vi "Stop Point.vi"(5 "Series Enqueuer":refnum<class "Message Enqueuer.lvclass">, 7 "Task-Point Ident":string, 8 "error in":errorcluster, 11 "MSS in":refnum<class "Measure and Stimulus Subsystems.lvclass">) -> (0 "error out":errorcluster, 3 "MSS out":refnum<class "Measure and Stimulus Subsystems.lvclass">)   [LabVIEW 2023, in "HAL GOOP4.lvlib" / "Measure and Stimulus Subsystems.lvclass"]
uses:
  Measure and Stimulus Subsystems.lvclass
  <vilib>/ActorFramework/Message Enqueuer/Message Enqueuer.lvclass
  Measure and Stimulus Subsystems.lvclass/Measure and Stimulus Subsystems.ctl
  Series/ISeries Actor/ISeries Actor Messages/Stop Point on Target Msg/Stop Point on Target Msg.lvclass/Stop Point on Target Msg.ctl
  <vilib>/ActorFramework/Message Enqueuer/Message Enqueuer.lvclass/Message Enqueuer.ctl
  <vilib>/ActorFramework/Message Enqueuer/Enqueue.vi
  Series/ISeries Actor/ISeries Actor Messages/Stop Point on Target Msg/Stop Point on Target Msg.lvclass
  <vilib>/Utility/LVClass/Get LV Class Name.vi
  <resource>/AFDebug/Generate Trace for Message.vi
  <vilib>/ActorFramework/Message Priority Queue/Priority Enqueue.vi
  Virt Instr Host/Virt Instr Local.lvclass
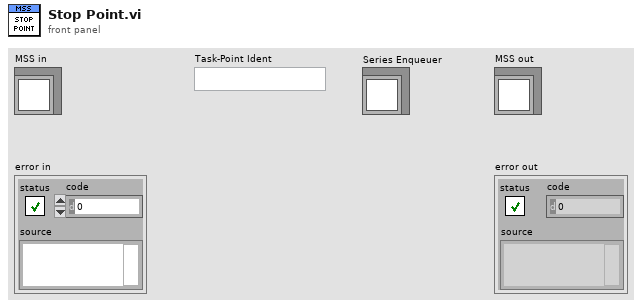
[diagram p1: front panel]
types:
  T1 = map{string, refnum<class "Virt Instr Local.lvclass">}
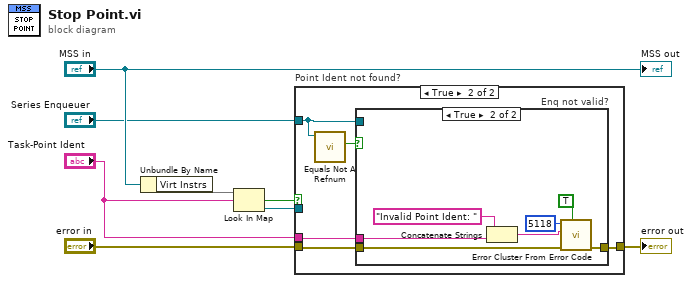
[diagram p0: block diagram]
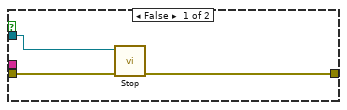
[diagram p2: hidden frame]
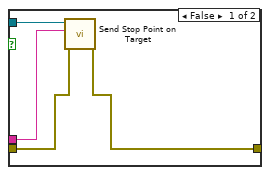
[diagram p3: hidden frame]
diagram:
  n1 = Unbundle By Name("MSS in") -> ("Virt Instrs"=w7:T1)
  n2 = Look In Map(map=w7, key="Task-Point Ident") -> (key not found?=w6:bool, value=w5:refnum<class "Virt Instr Local.lvclass">)  [unwired: 1 in]
  n3 = case "Point Ident not found?" shown="True" w6 {
    tunnel: w5 -> [w10 _]
    tunnel: "error in" -> [w9 w16]
    tunnel: [w11 w15] -> w4
    tunnel: "Series Enqueuer" -> [_ w12]
    tunnel: "Task-Point Ident" -> [_ w14]
    frame False {
      n4 = call-dynamic "Stop.vi"("error in (no error)"=w9, "Virt Instr Base in"=w10) -> ("error out"=w11:errorcluster)  [unwired: 8 in, 1 out]
    }
    frame True {
      n5 = call <vilib>:"Equals Not A Refnum.vi"("Message Enqueuer"=w12) -> ("Not a refnum?"=w13:bool)  [unwired: 10 in]
      n6 = case "Enq not valid?" shown="True" w13 {
        tunnel: w16 -> [w18 w23]
        tunnel: [w17 w22] -> w15
        tunnel: w14 -> [w19 w21]
        tunnel: w12 -> [w20 _]
        frame False {
          n7 = call "Send Stop Point on Target.vi"("error in (no error)"=w18, "Point Ident"=w19, "Message Enqueuer"=w20) -> ("error out"=w17:errorcluster)  [unwired: 7 in, 1 out]
        }
        frame True {
          n8 = Concatenate Strings("Invalid Point Ident: ", w21) -> (w25:string)
          n9 = call <vilib>:"Error Cluster From Error Code.vi"("show call chain? (False)"=TRUE, "error in (no error)"=w23, "error message (\"\")"=w25, "error code (0)"=5118) -> ("error out"=w22:errorcluster)  [unwired: 5 in]
        }
      }
    }
  }
  "error out" <- w4
  "MSS out" <- "MSS in"
